vi "SE_HV500.ProcCases.vi"(0 "i ref in":refnum<vi>, 1 "selector":string, 2 "Data":T1, 3 "call cluster":T2={"Object"="", "Selector"="", "CallType"=enum."synchronous", "Async Object"="", "Async Selector"="", "Data Descriptor"="", "Data"=[], "Error #"=0, "Expire"=0}, 5 "error in (no error)":errorcluster) -> (14 "i ref out":refnum<vi>, 17 "answer cluster":T2={"Object"="", "Selector"="", "CallType"=enum."synchronous", "Async Object"="", "Async Selector"="", "Data Descriptor"="", "Data"=[], "Error #"=0, "Expire"=0}, 19 "error out":errorcluster)   [LabVIEW 2014, in "SE_HV500.lvlib"]
doc: "This method is called by a process from within the default case in the event loop. The methods of a class that are linked to events will be called from THIS method. Add your code here."
uses:
  SE_HV500.lvlib
  CS_Core/CSSystem/CoreDefs/CoreDefs.call_type.ctl
  CS_Core/BaseProcess/BaseProcess.descriptor string definition.ctl
  CS_Core/CSSystem/CoreDefs/CoreDefs.rawDataType.ctl
  CS_Core/CSSystem/CoreLib/CoreLib.byte array 2 short.vi
  CS_Core/CSSystem/CoreLib/CoreLib.byte array 2 double.vi
  CS_Core/CSSystem/CoreLib/CoreLib.string 2 byte array.vi
  CS_Core/BaseProcess/BaseProcess.lvlib
  CS_Core/CSSystem/CoreLib/CoreLib.lvlib
  instr.lib/SE_HV500_Driver/SE_HV500Driver.lvlib
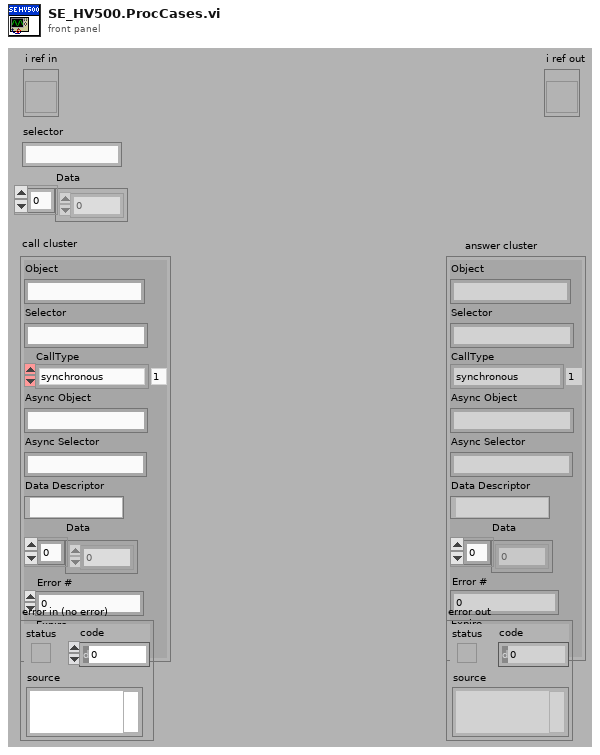
[diagram p1: front panel]
types:
  T1 = typedef "CoreDefs.rawDataType.ctl" = i8[]
  T2 = typedef "CoreDefs.call_type.ctl" = cluster{"Object":string, "Selector":string, "CallType":enum16{"simple", "synchronous", "asynchronous"}, "Async Object":string, "Async Selector":string, "Data Descriptor":T3, "Data":T1, "Error #":i32, "Expire":u32}
  T3 = typedef "BaseProcess.lvlib/BaseProcess.descriptor string definition.ctl" = string
  T4 = cluster{"CH 1":bool, "CH 2":bool, "CH 3":bool, "CH 4":bool, "CH 5":bool, "CH 6":bool, "CH 7":bool, "CH 8":bool, "CH 9":bool, "CH 10":bool, "CH 11":bool, "CH 12":bool, "CH 13":bool, "CH 14":bool, "CH 15":bool, "CH 16":bool}
  T5 = typedef "SE_HV500.lvlib/SE_HV500.i attribute.ctl" = cluster{"SetStatus":bool, "Set Voltage":dbl, "VoltageID":i32, "Nom Voltage":dbl, "VISA resource name in":refnum<visa-resource-name>, "Device name":string, "PSRange":i32}
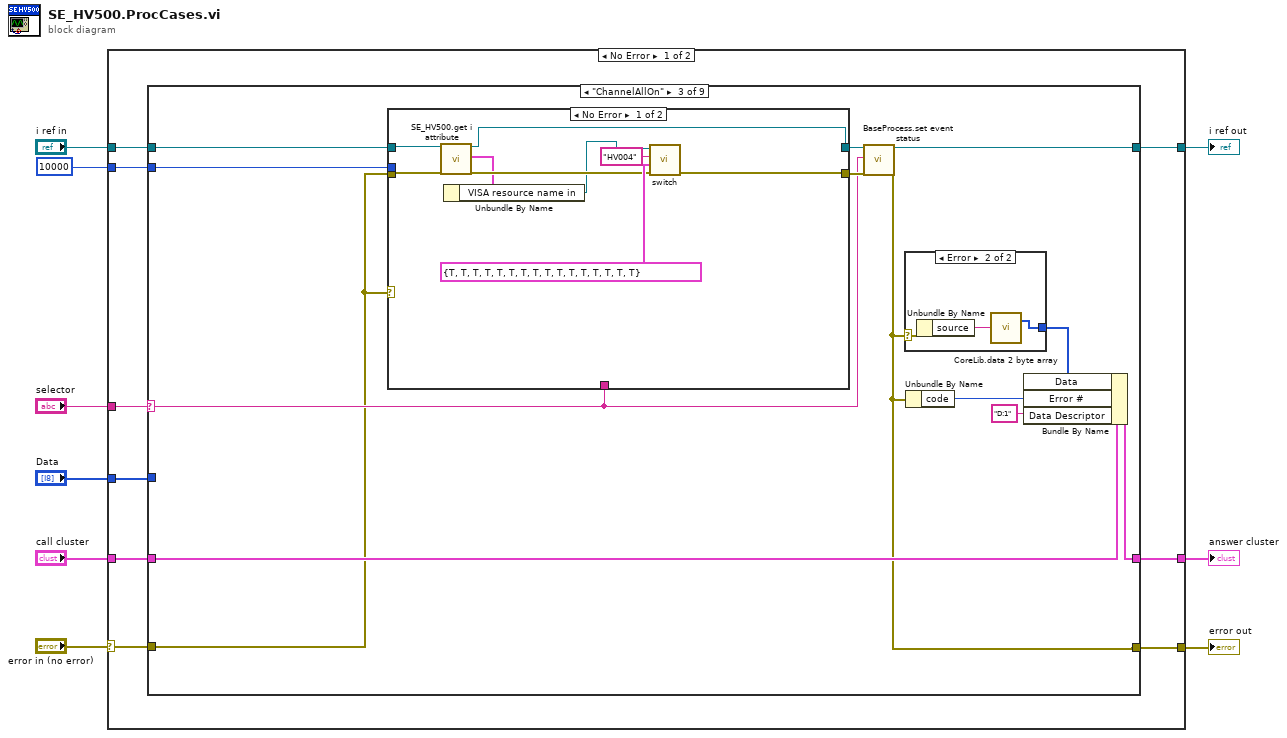
[diagram p0: block diagram]
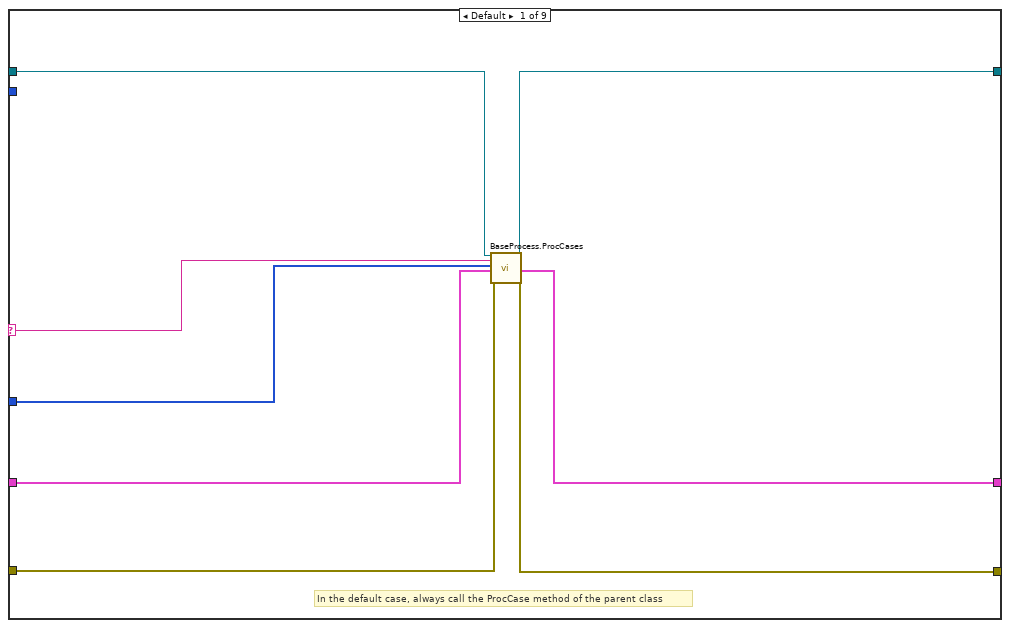
[diagram p2: hidden frame]
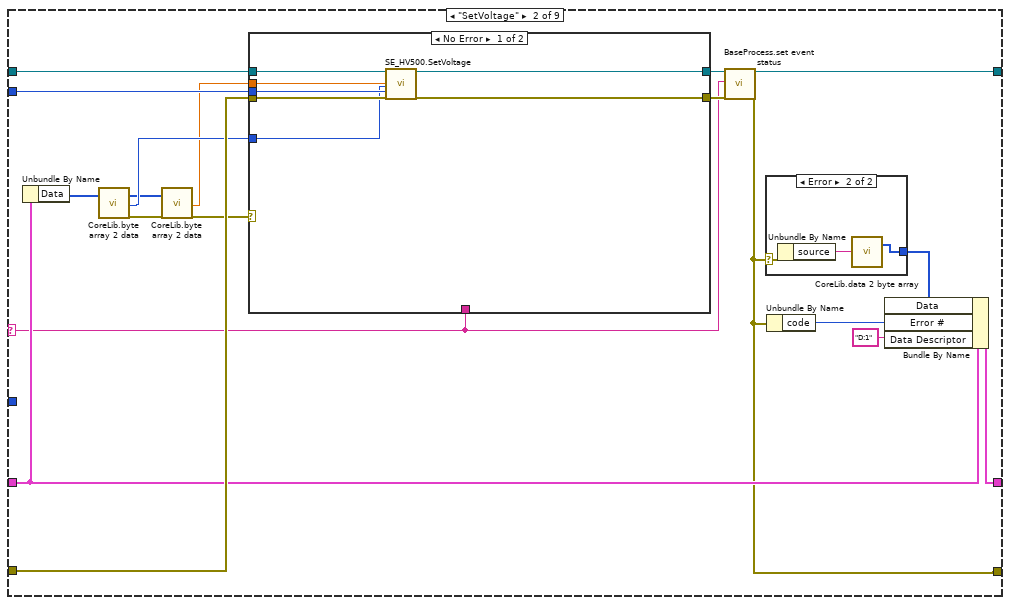
[diagram p3: hidden frame]
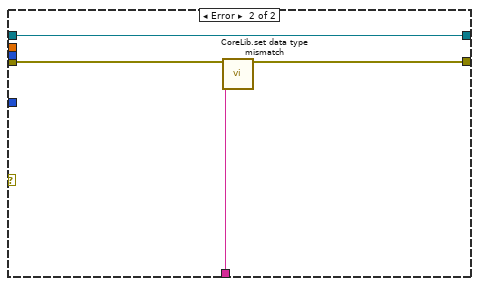
[diagram p5: hidden frame]
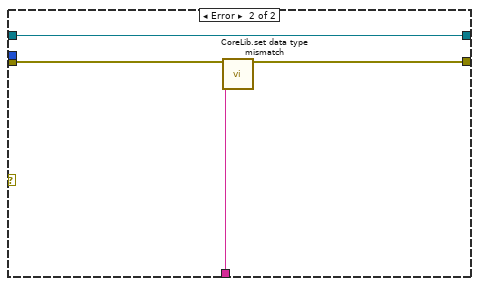
[diagram p7: hidden frame]
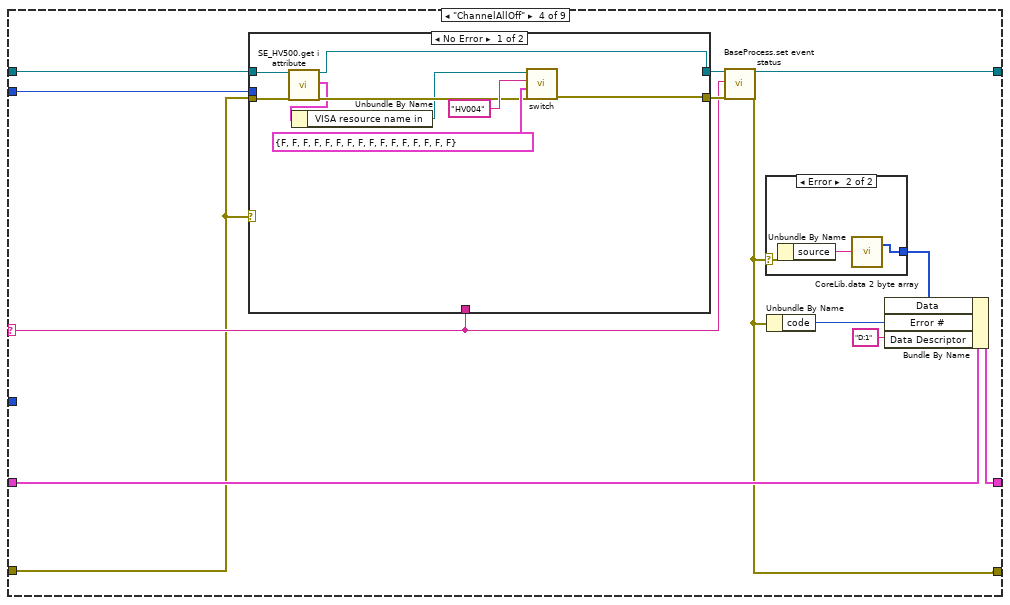
[diagram p8: hidden frame]
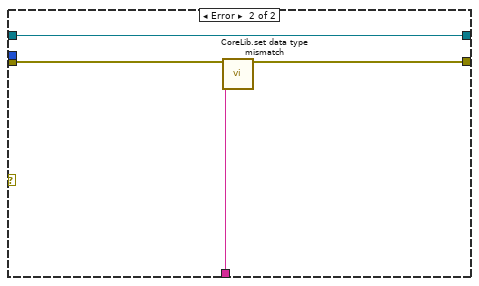
[diagram p10: hidden frame]
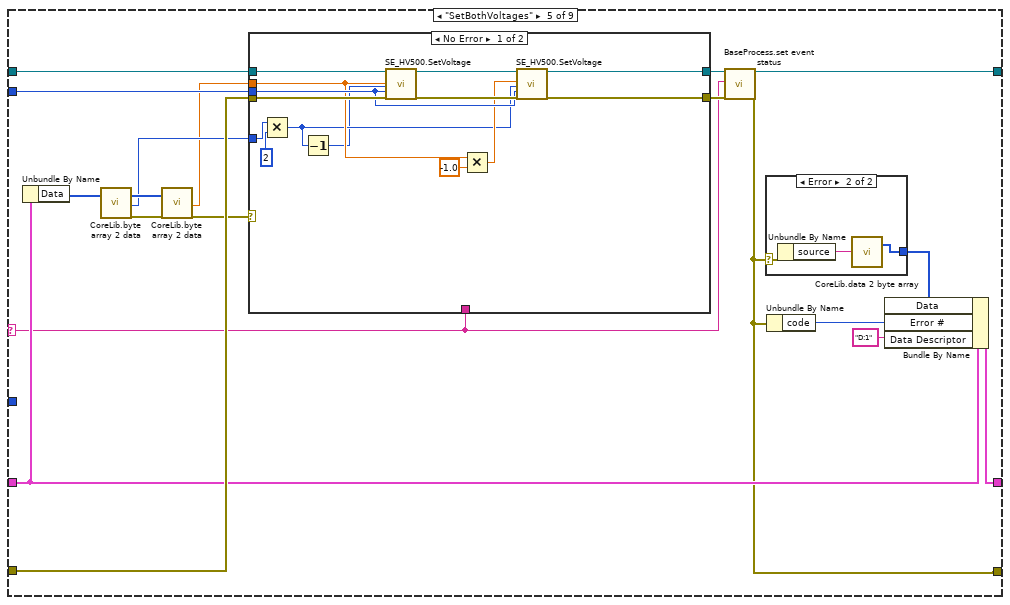
[diagram p11: hidden frame]
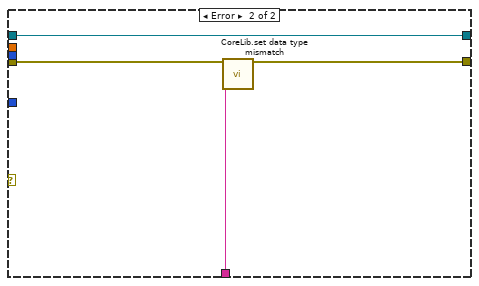
[diagram p13: hidden frame]
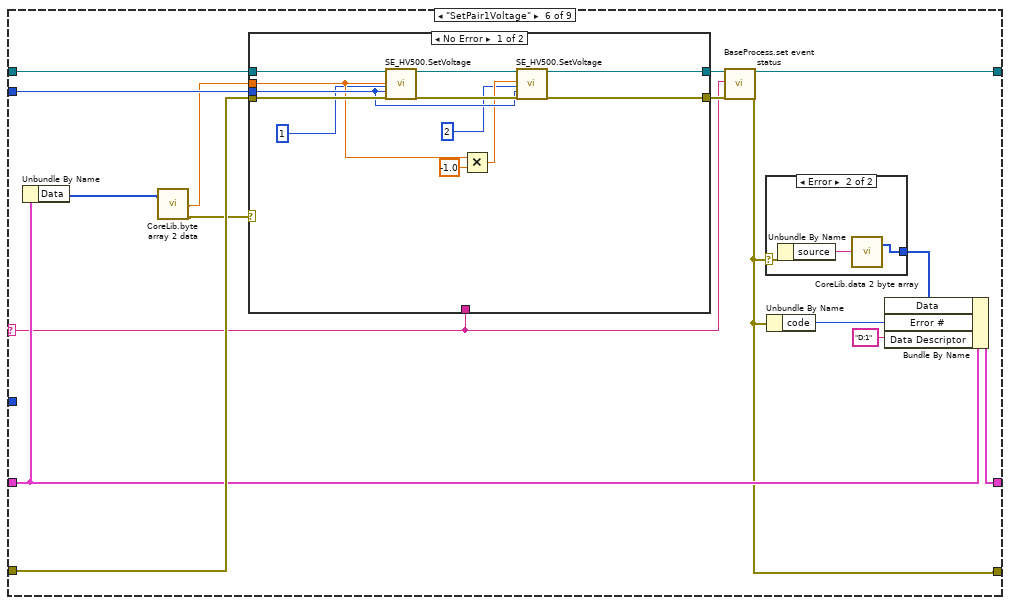
[diagram p14: hidden frame]
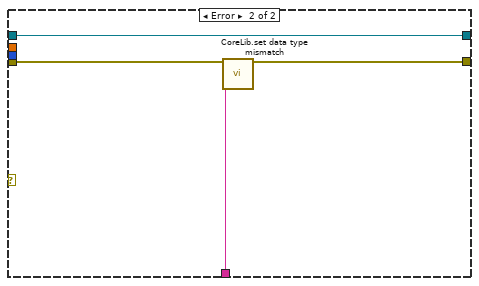
[diagram p16: hidden frame]
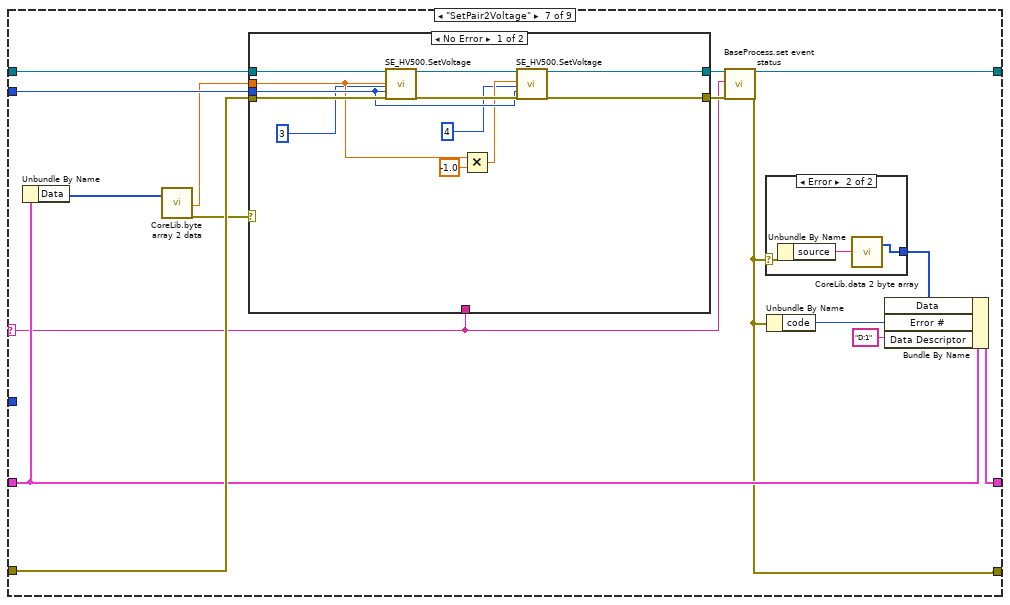
[diagram p17: hidden frame]
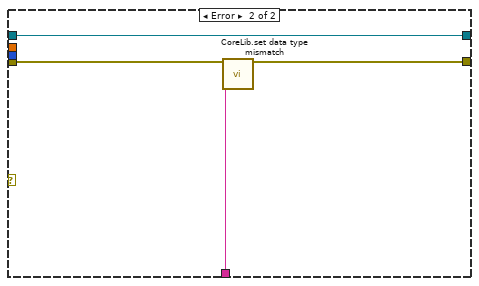
[diagram p19: hidden frame]
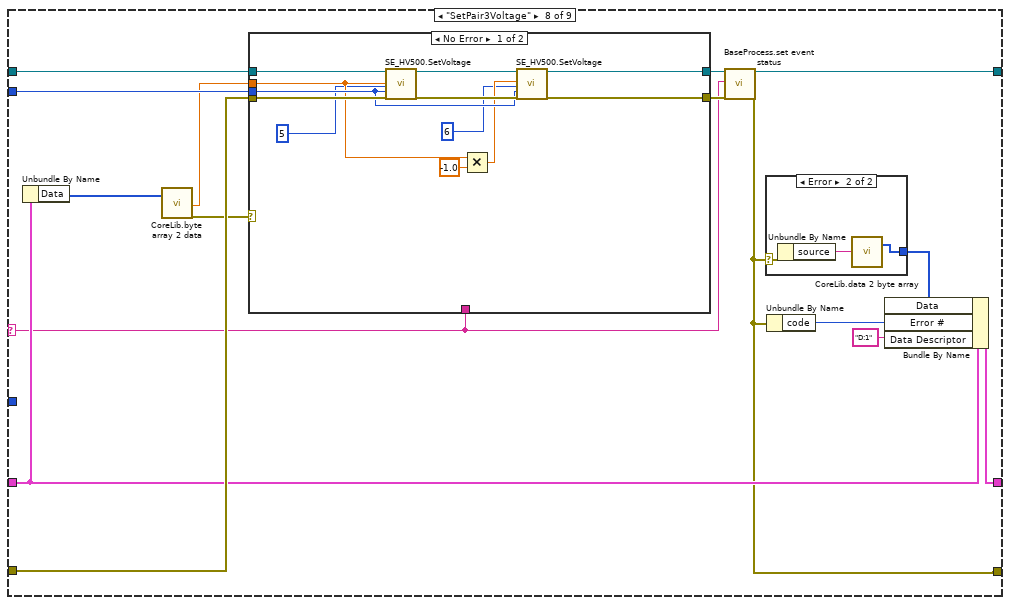
[diagram p20: hidden frame]
diagram:
  n1 = case shown="No Error" "error in (no error)" {
    selector: "error in (no error)" -> [w10 w298]
    tunnel: "selector" -> [w18 _]
    tunnel: [w17 w299] -> w8
    tunnel: "call cluster" -> [w16 w299]
    tunnel: "i ref in" -> [w15 w300]
    tunnel: [w14 w300] -> w5
    tunnel: [w13 w298] -> w4
    tunnel: 10000 -> [w12 _]
    tunnel: "Data" -> [w11 _]
    frame No Error {
      n2 = case shown="\"ChannelAllOn\"" w18 {
        selector: w18 -> [w20 w36 w64 w93 w127 w164 w199 w234 w269]
        tunnel: w11 -> [w21 _ _ _ _ _ _ _ _]
        tunnel: w15 -> [w19 w45 w72 w101 w136 w173 w208 w243 w278]
        tunnel: [w26 w35 w63 w92 w126 w163 w198 w233 w268] -> w14
        tunnel: w16 -> [w22 w42 w70 w99 w133 w170 w205 w240 w275]
        tunnel: [w23 w41 w69 w98 w132 w169 w204 w239 w274] -> w17
        tunnel: w10 -> [w25 w44 w60 w89 w135 w172 w207 w242 w277]
        tunnel: [w24 w37 w65 w94 w128 w165 w200 w235 w270] -> w13
        tunnel: w12 -> [_ w33 w61 w90 w124 w161 w196 w231 w266]
        frame Default {
          # "In the default case, always call the ProcCase method of the parent class"
          n3 = call "BaseProcess.ProcCases.vi"("i ref in"=w19, "selector"=w20, "Data"=w21, "call cluster"=w22, "error in (no error)"=w25) -> ("i ref out"=w26:refnum<vi>, "answer cluster"=w23:T2, "error out"=w24:errorcluster)  [unwired: 12 in]
        }
        frame "SetVoltage" {
          n4 = Unbundle By Name(w42) -> ("Data"=w32:T1)
          n5 = call-poly "CoreLib.byte array 2 data.vi"("byteArray"=w32) -> ("byteArray out"=w28:T1, "i16"=w31:i16, "error out"=w29:errorcluster)  [unwired: 16 in]
          n6 = call-poly "CoreLib.byte array 2 data.vi"("byteArray"=w28, "error in (no error)"=w29) -> ("d64"=w27:dbl, "error out"=w30:errorcluster)  [unwired: 15 in, 1 out]
          n7 = case shown="No Error" w30 {
            tunnel: [w50 w59] -> w39
            tunnel: w45 -> [w54 w59]
            tunnel: w44 -> [w55 w58]
            tunnel: [w51 w57] -> w38
            tunnel: w36 -> [_ w56]
            tunnel: w27 -> [w53 _]
            tunnel: w33 -> [w52 _]
            tunnel: w31 -> [w49 _]
            frame No Error {
              n8 = call "SE_HV500.SetVoltage.vi"("i ref in"=w54, "Set Voltage"=w53, "Channel"=w49, "Time out"=w52, "error in (no error)"=w55) -> ("i ref out"=w50:refnum<vi>, "error out"=w51:errorcluster)  [unwired: 12 in, 1 out]
            }
            frame Error {
              n9 = call "CoreLib.set data type mismatch.vi"("error in (no error)"=w58, "error source"=w56) -> ("error out"=w57:errorcluster)  [unwired: 17 in]
            }
          }
          n10 = call "BaseProcess.set event status.vi"("i ref in"=w39, "EventStatus"=w36, "error in (no error)"=w38) -> ("i ref out"=w35:refnum<vi>, "error out"=w37:errorcluster)  [unwired: 14 in, 1 out]
          n11 = case shown="Error" w37 {
            selector: w37 -> [_ w48]
            tunnel: [_ w46] -> w40
            frame No Error {
            }
            frame Error {
              n12 = Unbundle By Name(w48) -> ("source"=w47:string)
              n13 = call-poly "CoreLib.data 2 byte array.vi"("string"=w47) -> ("byteArray out"=w46:T1)  [unwired: 18 in]
            }
          }
          n14 = Unbundle By Name(w37) -> ("code"=w43:i32)
          n15 = Bundle By Name(cluster=w42, "Data"=w40, "Error #"=w43, "Data Descriptor"="D:1") -> (w41:T2)
        }
        frame "ChannelAllOn" {
          n16 = case shown="No Error" w60 {
            tunnel: [w79 w88] -> w67
            tunnel: w72 -> [w80 w88]
            tunnel: w60 -> [w81 w87]
            tunnel: [w84 w86] -> w66
            tunnel: w64 -> [_ w85]
            tunnel: w61 -> [_ _]
            frame No Error {
              n17 = call "SE_HV500.get i attribute.vi"("i ref in"=w80, "error in (no error)"=w81) -> ("i ref out"=w79:refnum<vi>, "i attribute"=w77:T5, "error out"=w78:errorcluster)  [unwired: 15 in]
              n18 = Unbundle By Name(w77) -> ("VISA resource name in"=w76:refnum<visa-resource-name>)
              n19 = call "switch.vi"("Error in"=w78, "Inputs"=T4 {"CH 1"=TRUE, "CH 2"=TRUE, "CH 3"=TRUE, "CH 4"=TRUE, "CH 5"=TRUE, "CH 6"=TRUE, "CH 7"=TRUE, "CH 8"=TRUE, "CH 9"=TRUE, "CH 10"=TRUE, "CH 11"=TRUE, "CH 12"=TRUE, "CH 13"=TRUE, "CH 14"=TRUE, "CH 15"=TRUE, "CH 16"=TRUE}, "Device name"="HV004", "VISA resource name in"=w76) -> ("Error out"=w84:errorcluster)  [unwired: 6 in, 1 out]
            }
            frame Error {
              n20 = call "CoreLib.set data type mismatch.vi"("error in (no error)"=w87, "error source"=w85) -> ("error out"=w86:errorcluster)  [unwired: 17 in]
            }
          }
          n21 = call "BaseProcess.set event status.vi"("i ref in"=w67, "EventStatus"=w64, "error in (no error)"=w66) -> ("i ref out"=w63:refnum<vi>, "error out"=w65:errorcluster)  [unwired: 14 in, 1 out]
          n22 = case shown="Error" w65 {
            selector: w65 -> [_ w75]
            tunnel: [_ w73] -> w68
            frame No Error {
            }
            frame Error {
              n23 = Unbundle By Name(w75) -> ("source"=w74:string)
              n24 = call-poly "CoreLib.data 2 byte array.vi"("string"=w74) -> ("byteArray out"=w73:T1)  [unwired: 18 in]
            }
          }
          n25 = Unbundle By Name(w65) -> ("code"=w71:i32)
          n26 = Bundle By Name(cluster=w70, "Data"=w68, "Error #"=w71, "Data Descriptor"="D:1") -> (w69:T2)
        }
        frame "ChannelAllOff" {
          n27 = case shown="No Error" w89 {
            tunnel: [w107 w117] -> w96
            tunnel: w101 -> [w108 w117]
            tunnel: w89 -> [w110 w116]
            tunnel: [w113 w115] -> w95
            tunnel: w93 -> [_ w114]
            tunnel: w90 -> [_ _]
            frame No Error {
              n28 = call "SE_HV500.get i attribute.vi"("i ref in"=w108, "error in (no error)"=w110) -> ("i ref out"=w107:refnum<vi>, "i attribute"=w105:T5, "error out"=w109:errorcluster)  [unwired: 15 in]
              n29 = Unbundle By Name(w105) -> ("VISA resource name in"=w106:refnum<visa-resource-name>)
              n30 = call "switch.vi"("Error in"=w109, "Inputs"=T4 {"CH 1"=FALSE, "CH 2"=FALSE, "CH 3"=FALSE, "CH 4"=FALSE, "CH 5"=FALSE, "CH 6"=FALSE, "CH 7"=FALSE, "CH 8"=FALSE, "CH 9"=FALSE, "CH 10"=FALSE, "CH 11"=FALSE, "CH 12"=FALSE, "CH 13"=FALSE, "CH 14"=FALSE, "CH 15"=FALSE, "CH 16"=FALSE}, "Device name"="HV004", "VISA resource name in"=w106) -> ("Error out"=w113:errorcluster)  [unwired: 6 in, 1 out]
            }
            frame Error {
              n31 = call "CoreLib.set data type mismatch.vi"("error in (no error)"=w116, "error source"=w114) -> ("error out"=w115:errorcluster)  [unwired: 17 in]
            }
          }
          n32 = call "BaseProcess.set event status.vi"("i ref in"=w96, "EventStatus"=w93, "error in (no error)"=w95) -> ("i ref out"=w92:refnum<vi>, "error out"=w94:errorcluster)  [unwired: 14 in, 1 out]
          n33 = case shown="Error" w94 {
            selector: w94 -> [_ w104]
            tunnel: [_ w102] -> w97
            frame No Error {
            }
            frame Error {
              n34 = Unbundle By Name(w104) -> ("source"=w103:string)
              n35 = call-poly "CoreLib.data 2 byte array.vi"("string"=w103) -> ("byteArray out"=w102:T1)  [unwired: 18 in]
            }
          }
          n36 = Unbundle By Name(w94) -> ("code"=w100:i32)
          n37 = Bundle By Name(cluster=w99, "Data"=w97, "Error #"=w100, "Data Descriptor"="D:1") -> (w98:T2)
        }
        frame "SetBothVoltages" {
          n38 = Unbundle By Name(w133) -> ("Data"=w123:T1)
          n39 = call-poly "CoreLib.byte array 2 data.vi"("byteArray"=w123) -> ("byteArray out"=w122:T1, "i16"=w119:i16, "error out"=w120:errorcluster)  [unwired: 16 in]
          n40 = call-poly "CoreLib.byte array 2 data.vi"("byteArray"=w122, "error in (no error)"=w120) -> ("d64"=w118:dbl, "error out"=w121:errorcluster)  [unwired: 15 in, 1 out]
          n41 = case shown="No Error" w121 {
            tunnel: [w148 w157] -> w130
            tunnel: w136 -> [w152 w157]
            tunnel: w135 -> [w153 w156]
            tunnel: [w150 w155] -> w129
            tunnel: w127 -> [_ w154]
            tunnel: w118 -> [w144 _]
            tunnel: w124 -> [w146 _]
            tunnel: w119 -> [w141 _]
            frame No Error {
              n42 = Multiply(x=w141, y=i16 2) -> (x*y=w142:i16)
              n43 = Decrement(x=w142) -> (x-1=w140:i16)
              n44 = call "SE_HV500.SetVoltage.vi"("i ref in"=w152, "Set Voltage"=w144, "Channel"=w140, "Time out"=w146, "error in (no error)"=w153) -> ("i ref out"=w149:refnum<vi>, "error out"=w151:errorcluster)  [unwired: 12 in, 1 out]
              n45 = Multiply(x=w144, y=-1.0) -> (x*y=w143:dbl)
              n46 = call "SE_HV500.SetVoltage.vi"("i ref in"=w149, "Set Voltage"=w143, "Channel"=w142, "Time out"=w146, "error in (no error)"=w151) -> ("i ref out"=w148:refnum<vi>, "error out"=w150:errorcluster)  [unwired: 12 in, 1 out]
            }
            frame Error {
              n47 = call "CoreLib.set data type mismatch.vi"("error in (no error)"=w156, "error source"=w154) -> ("error out"=w155:errorcluster)  [unwired: 17 in]
            }
          }
          n48 = call "BaseProcess.set event status.vi"("i ref in"=w130, "EventStatus"=w127, "error in (no error)"=w129) -> ("i ref out"=w126:refnum<vi>, "error out"=w128:errorcluster)  [unwired: 14 in, 1 out]
          n49 = case shown="Error" w128 {
            selector: w128 -> [_ w139]
            tunnel: [_ w137] -> w131
            frame No Error {
            }
            frame Error {
              n50 = Unbundle By Name(w139) -> ("source"=w138:string)
              n51 = call-poly "CoreLib.data 2 byte array.vi"("string"=w138) -> ("byteArray out"=w137:T1)  [unwired: 18 in]
            }
          }
          n52 = Unbundle By Name(w128) -> ("code"=w134:i32)
          n53 = Bundle By Name(cluster=w133, "Data"=w131, "Error #"=w134, "Data Descriptor"="D:1") -> (w132:T2)
        }
        frame "SetPair1Voltage" {
          n54 = Unbundle By Name(w170) -> ("Data"=w159:T1)
          n55 = call-poly "CoreLib.byte array 2 data.vi"("byteArray"=w159) -> ("d64"=w158:dbl, "error out"=w160:errorcluster)  [unwired: 16 in, 1 out]
          n56 = case shown="No Error" w160 {
            tunnel: [w183 w192] -> w167
            tunnel: w173 -> [w187 w192]
            tunnel: w172 -> [w188 w191]
            tunnel: [w185 w190] -> w166
            tunnel: w164 -> [_ w189]
            tunnel: w158 -> [w180 _]
            tunnel: w161 -> [w182 _]
            frame No Error {
              n57 = call "SE_HV500.SetVoltage.vi"("i ref in"=w187, "Set Voltage"=w180, "Channel"=i16 1, "Time out"=w182, "error in (no error)"=w188) -> ("i ref out"=w184:refnum<vi>, "error out"=w186:errorcluster)  [unwired: 12 in, 1 out]
              n58 = Multiply(x=w180, y=-1.0) -> (x*y=w179:dbl)
              n59 = call "SE_HV500.SetVoltage.vi"("i ref in"=w184, "Set Voltage"=w179, "Channel"=i16 2, "Time out"=w182, "error in (no error)"=w186) -> ("i ref out"=w183:refnum<vi>, "error out"=w185:errorcluster)  [unwired: 12 in, 1 out]
            }
            frame Error {
              n60 = call "CoreLib.set data type mismatch.vi"("error in (no error)"=w191, "error source"=w189) -> ("error out"=w190:errorcluster)  [unwired: 17 in]
            }
          }
          n61 = call "BaseProcess.set event status.vi"("i ref in"=w167, "EventStatus"=w164, "error in (no error)"=w166) -> ("i ref out"=w163:refnum<vi>, "error out"=w165:errorcluster)  [unwired: 14 in, 1 out]
          n62 = case shown="Error" w165 {
            selector: w165 -> [_ w176]
            tunnel: [_ w174] -> w168
            frame No Error {
            }
            frame Error {
              n63 = Unbundle By Name(w176) -> ("source"=w175:string)
              n64 = call-poly "CoreLib.data 2 byte array.vi"("string"=w175) -> ("byteArray out"=w174:T1)  [unwired: 18 in]
            }
          }
          n65 = Unbundle By Name(w165) -> ("code"=w171:i32)
          n66 = Bundle By Name(cluster=w170, "Data"=w168, "Error #"=w171, "Data Descriptor"="D:1") -> (w169:T2)
        }
        frame "SetPair2Voltage" {
          n67 = Unbundle By Name(w205) -> ("Data"=w194:T1)
          n68 = call-poly "CoreLib.byte array 2 data.vi"("byteArray"=w194) -> ("d64"=w193:dbl, "error out"=w195:errorcluster)  [unwired: 16 in, 1 out]
          n69 = case shown="No Error" w195 {
            tunnel: [w218 w227] -> w202
            tunnel: w208 -> [w222 w227]
            tunnel: w207 -> [w223 w226]
            tunnel: [w220 w225] -> w201
            tunnel: w199 -> [_ w224]
            tunnel: w193 -> [w215 _]
            tunnel: w196 -> [w217 _]
            frame No Error {
              n70 = call "SE_HV500.SetVoltage.vi"("i ref in"=w222, "Set Voltage"=w215, "Channel"=i16 3, "Time out"=w217, "error in (no error)"=w223) -> ("i ref out"=w219:refnum<vi>, "error out"=w221:errorcluster)  [unwired: 12 in, 1 out]
              n71 = Multiply(x=w215, y=-1.0) -> (x*y=w214:dbl)
              n72 = call "SE_HV500.SetVoltage.vi"("i ref in"=w219, "Set Voltage"=w214, "Channel"=i16 4, "Time out"=w217, "error in (no error)"=w221) -> ("i ref out"=w218:refnum<vi>, "error out"=w220:errorcluster)  [unwired: 12 in, 1 out]
            }
            frame Error {
              n73 = call "CoreLib.set data type mismatch.vi"("error in (no error)"=w226, "error source"=w224) -> ("error out"=w225:errorcluster)  [unwired: 17 in]
            }
          }
          n74 = call "BaseProcess.set event status.vi"("i ref in"=w202, "EventStatus"=w199, "error in (no error)"=w201) -> ("i ref out"=w198:refnum<vi>, "error out"=w200:errorcluster)  [unwired: 14 in, 1 out]
          n75 = case shown="Error" w200 {
            selector: w200 -> [_ w211]
            tunnel: [_ w209] -> w203
            frame No Error {
            }
            frame Error {
              n76 = Unbundle By Name(w211) -> ("source"=w210:string)
              n77 = call-poly "CoreLib.data 2 byte array.vi"("string"=w210) -> ("byteArray out"=w209:T1)  [unwired: 18 in]
            }
          }
          n78 = Unbundle By Name(w200) -> ("code"=w206:i32)
          n79 = Bundle By Name(cluster=w205, "Data"=w203, "Error #"=w206, "Data Descriptor"="D:1") -> (w204:T2)
        }
        frame "SetPair3Voltage" {
          n80 = Unbundle By Name(w240) -> ("Data"=w229:T1)
          n81 = call-poly "CoreLib.byte array 2 data.vi"("byteArray"=w229) -> ("d64"=w228:dbl, "error out"=w230:errorcluster)  [unwired: 16 in, 1 out]
          n82 = case shown="No Error" w230 {
            tunnel: [w253 w262] -> w237
            tunnel: w243 -> [w257 w262]
            tunnel: w242 -> [w258 w261]
            tunnel: [w255 w260] -> w236
            tunnel: w234 -> [_ w259]
            tunnel: w228 -> [w250 _]
            tunnel: w231 -> [w252 _]
            frame No Error {
              n83 = call "SE_HV500.SetVoltage.vi"("i ref in"=w257, "Set Voltage"=w250, "Channel"=i16 5, "Time out"=w252, "error in (no error)"=w258) -> ("i ref out"=w254:refnum<vi>, "error out"=w256:errorcluster)  [unwired: 12 in, 1 out]
              n84 = Multiply(x=w250, y=-1.0) -> (x*y=w249:dbl)
              n85 = call "SE_HV500.SetVoltage.vi"("i ref in"=w254, "Set Voltage"=w249, "Channel"=i16 6, "Time out"=w252, "error in (no error)"=w256) -> ("i ref out"=w253:refnum<vi>, "error out"=w255:errorcluster)  [unwired: 12 in, 1 out]
            }
            frame Error {
              n86 = call "CoreLib.set data type mismatch.vi"("error in (no error)"=w261, "error source"=w259) -> ("error out"=w260:errorcluster)  [unwired: 17 in]
            }
          }
          n87 = call "BaseProcess.set event status.vi"("i ref in"=w237, "EventStatus"=w234, "error in (no error)"=w236) -> ("i ref out"=w233:refnum<vi>, "error out"=w235:errorcluster)  [unwired: 14 in, 1 out]
          n88 = case shown="Error" w235 {
            selector: w235 -> [_ w246]
            tunnel: [_ w244] -> w238
            frame No Error {
            }
            frame Error {
              n89 = Unbundle By Name(w246) -> ("source"=w245:string)
              n90 = call-poly "CoreLib.data 2 byte array.vi"("string"=w245) -> ("byteArray out"=w244:T1)  [unwired: 18 in]
            }
          }
          n91 = Unbundle By Name(w235) -> ("code"=w241:i32)
          n92 = Bundle By Name(cluster=w240, "Data"=w238, "Error #"=w241, "Data Descriptor"="D:1") -> (w239:T2)
        }
        frame "SetPair4Voltage" {
          n93 = Unbundle By Name(w275) -> ("Data"=w264:T1)
          n94 = call-poly "CoreLib.byte array 2 data.vi"("byteArray"=w264) -> ("d64"=w263:dbl, "error out"=w265:errorcluster)  [unwired: 16 in, 1 out]
          n95 = case shown="No Error" w265 {
            tunnel: [w288 w297] -> w272
            tunnel: w278 -> [w292 w297]
            tunnel: w277 -> [w293 w296]
            tunnel: [w290 w295] -> w271
            tunnel: w269 -> [_ w294]
            tunnel: w263 -> [w285 _]
            tunnel: w266 -> [w287 _]
            frame No Error {
              n96 = call "SE_HV500.SetVoltage.vi"("i ref in"=w292, "Set Voltage"=w285, "Channel"=i16 7, "Time out"=w287, "error in (no error)"=w293) -> ("i ref out"=w289:refnum<vi>, "error out"=w291:errorcluster)  [unwired: 12 in, 1 out]
              n97 = Multiply(x=w285, y=-1.0) -> (x*y=w284:dbl)
              n98 = call "SE_HV500.SetVoltage.vi"("i ref in"=w289, "Set Voltage"=w284, "Channel"=i16 8, "Time out"=w287, "error in (no error)"=w291) -> ("i ref out"=w288:refnum<vi>, "error out"=w290:errorcluster)  [unwired: 12 in, 1 out]
            }
            frame Error {
              n99 = call "CoreLib.set data type mismatch.vi"("error in (no error)"=w296, "error source"=w294) -> ("error out"=w295:errorcluster)  [unwired: 17 in]
            }
          }
          n100 = call "BaseProcess.set event status.vi"("i ref in"=w272, "EventStatus"=w269, "error in (no error)"=w271) -> ("i ref out"=w268:refnum<vi>, "error out"=w270:errorcluster)  [unwired: 14 in, 1 out]
          n101 = case shown="Error" w270 {
            selector: w270 -> [_ w281]
            tunnel: [_ w279] -> w273
            frame No Error {
            }
            frame Error {
              n102 = Unbundle By Name(w281) -> ("source"=w280:string)
              n103 = call-poly "CoreLib.data 2 byte array.vi"("string"=w280) -> ("byteArray out"=w279:T1)  [unwired: 18 in]
            }
          }
          n104 = Unbundle By Name(w270) -> ("code"=w276:i32)
          n105 = Bundle By Name(cluster=w275, "Data"=w273, "Error #"=w276, "Data Descriptor"="D:1") -> (w274:T2)
        }
      }
    }
    frame Error {
    }
  }
  "answer cluster" <- w8
  "i ref out" <- w5
  "error out" <- w4
